vi "Error_EnqueueError.vi"(7 "SourcePath":path, 9 "Error in":errorcluster, 10 "Message":string) -> (1 "error out":errorcluster)   [LabVIEW 2016]
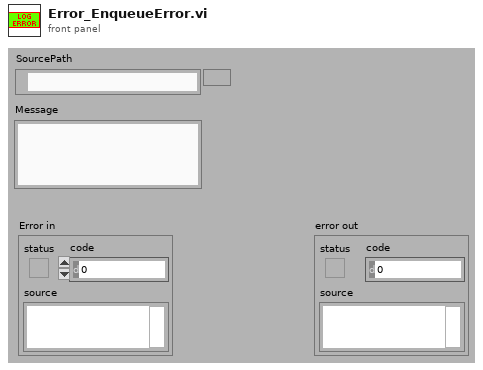
[diagram p1: front panel]
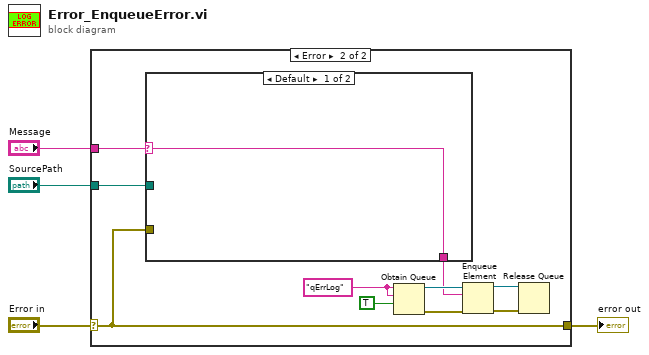
[diagram p0: block diagram]
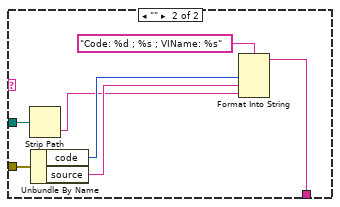
[diagram p3: hidden frame]
diagram:
  n1 = case shown="Error" "Error in" {
    selector: "Error in" -> [w5 w9]
    tunnel: [w5 w9] -> w3
    tunnel: "Message" -> [_ w6]
    tunnel: "SourcePath" -> [_ w7]
    frame No Error {
    }
    frame Error {
      w15 = "qErrLog" ("name (unnamed)")
      n2 = case shown="Default" w6 {
        selector: w6 -> [w16 _]
        tunnel: w9 -> [_ w22]
        tunnel: [w16 w20] -> w8
        tunnel: w7 -> [_ w18]
        frame Default {
        }
        frame "" {
          n3 = Strip Path(path=w18) -> (name=w17:string)  [unwired: 1 out]
          n4 = Unbundle By Name(w22) -> ("code"=w19:i32, "source"=w23:string)
          n5 = Format Into String(format string="Code: %d ; %s ; VIName: %s", w19, w23, w17) -> (resulting string=w20:string)  [unwired: 2 in, 1 out]
        }
      }
      n6 = Obtain Queue(name (unnamed)=w15, element data type=w15, create if not found? (T)=TRUE) -> (queue out=w14:refnum<queue>, error out=w13:errorcluster)  [unwired: 2 in, 1 out]
      n7 = Enqueue Element(queue=w14, element=w8, error in (no error)=w13) -> (queue out=w12:refnum<queue>, error out=w11:errorcluster)  [unwired: 2 out]
      n8 = Release Queue(queue=w12, error in (no error)=w11) -> ()  [unwired: 4 out]
    }
  }
  "error out" <- w3
